vi "WriteAO.vi"(8 "error in (no error)":errorcluster, 10 "AO_writeValue":dbl, 11 "FPGA VI Reference In":refnum<k20>) -> (0 "error out":errorcluster, 3 "FPGA VI Reference Out":refnum<k20>)   [LabVIEW 2020, in "FPGA_IO.lvlib"]
doc: "Write AO values in the FPGA\nChannels: C/AO0"
uses:
  FPGA_IO.lvlib
  <vilib>/Utility/error.llb/Error Cluster From Error Code.vi
  <vilib>/rvi/errors/niLvFpgaAdjustHostInterfaceError.vi
  <vilib>/rvi/interface/nirviReadWriteControl/nirviReadWriteControl.xnode
  NiFpgaLv.dll
  <vilib>/rvi/interface/Simulation/niFpgaSimulationCallBeginRW.vi
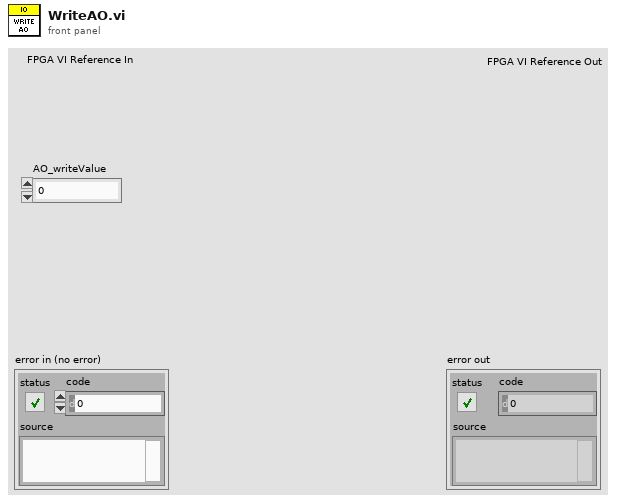
[diagram p1: front panel]
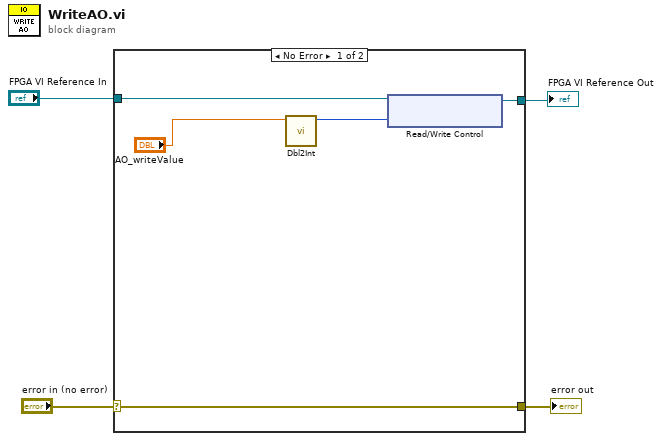
[diagram p0: block diagram]
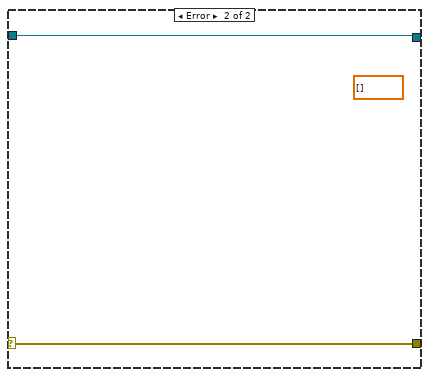
[diagram p2: hidden frame]
diagram:
  n1 = case shown="No Error" "error in (no error)" {
    selector: "error in (no error)" -> [w7 w10]
    tunnel: "FPGA VI Reference In" -> [w9 w11]
    tunnel: [w8 w11] -> w3
    tunnel: [w7 w10] -> w1
    frame No Error {
      n2 = call "Dbl2Int.vi"("AO_converted [V]"="AO_writeValue") -> ("AO_raw"=w5:i16)  [unwired: 10 in]
      n3 = xnode "Read/Write Control"("FPGA VI Reference In"=w9, "C_AO0_writeValue"=w5) -> ("FPGA VI Reference Out"=w8:refnum<k20>)  [unwired: 1 in, 1 out]
    }
    frame Error {
      (unwired) dbl[] []
    }
  }
  "FPGA VI Reference Out" <- w3
  "error out" <- w1
